vi "Extract Hex Number.vi"(10 "index":i32, 11 "unsigned byte array":u8[](array[numeric])) -> (3 "Numeric":u16)   [LabVIEW 2015]
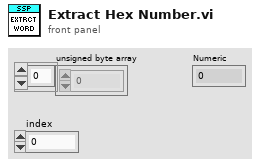
[diagram p1: front panel]
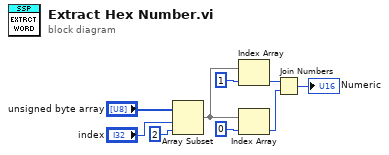
[diagram p0: block diagram]
diagram:
  n1 = Array Subset(array="unsigned byte array", index="index", length=2) -> (w5:u8[])
  n2 = Index Array(array=w5, index=1) -> (element=w7:u8)
  n3 = Index Array(array=w5, index=0) -> (element=w8:u8)
  n4 = Join Numbers(hi=w7, lo=w8) -> ((hi.lo)=→"Numeric":u16)
